vi "test message before initialize.vi"() -> ()   [LabVIEW 2017]
uses:
  user.lib/_NEVSTOP/Communicable State Machine(CSM)/Communicable State Machine.lvlib
panel:
  out "VIREF":string
  out "error out":errorcluster
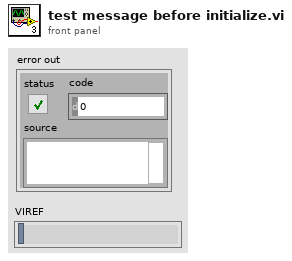
[diagram p1: front panel]
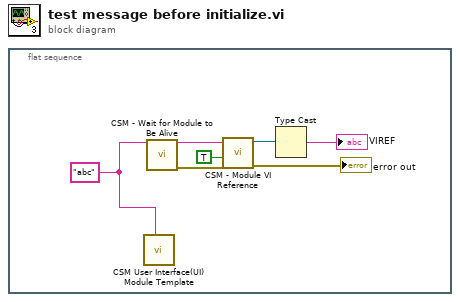
[diagram p0: block diagram]
diagram:
  n1 = flat-sequence {
    frame #0 {
      w2 = "abc" ("Name(\"\" to use uuid)")
      n2 = call "CSM User Interface(UI) Module Template.vi"("Name(\"\" to use uuid)"=w2) -> ()  [unwired: 11 in]
      n3 = call "CSM - Wait for Module to Be Alive.vi"("CSM Name"=w2) -> ("CSM Name(dup)"=w3:string, "error out"=w1:errorcluster)  [unwired: 12 in, 1 out]
      n4 = call "CSM - Module VI Reference.vi"("error in (no error)"=w1, "force?(F)"=TRUE, "CSM Name"=w3) -> ("error out"=→"error out":errorcluster, "CSM Module VIRef"=w5:refnum<vi>)  [unwired: 7 in]
      n5 = Type Cast(x=w5) -> (*(type *) &x=→"VIREF":string)  [unwired: 1 in]
    }
  }
